vi "Yokogawa WT300 Series Measure Harmonics Preset.vi"() -> ()   [LabVIEW 2016]
doc: "This example shows how to measure the harmonic measurement numeric preset list data\n\n<b>Note:</b>\nThis setting valid on models with the harmonic measurement (/G5) option."
uses:
  Public/Data/Read Measurement (Harmonics).vi
  Yokogawa WT300 Series.lvlib
panel:
  in  "Preset (1:Pattern 1)":i32(ring)=1 items=["Pattern 1"=1, "Pattern 2"=2, "Pattern 3"=3, "Pattern 4"=4]
  out "Measurement":dbl[][](array[numeric])
  out "Function":string[](array[string])
  in  "Number of Item (15)":i32=15 min=1 max=32
  in  "Timeout (10000 ms)":i32=10000 min=1
  in  "VISA resource name":refnum<visa-resource-name>
  # "(c) 2013 Yokogawa Meters & Instruments Corporation.  All rights reserved."
  # "WT300 SERIES POWER ANALYZER"
  # "Total        DC            1             2              3             4"
  # "ms"
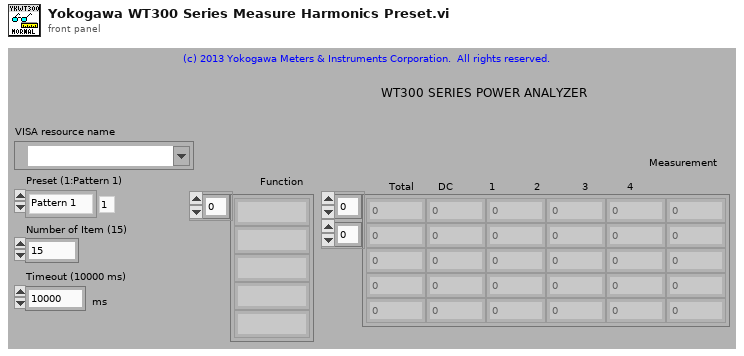
[diagram p1: front panel]
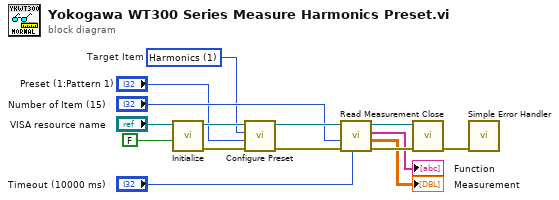
[diagram p0: block diagram]
diagram:
  w2 = 1 items=["Normal", "Harmonics"]  # Target Item
  n1 = call "Initialize.vi"("Reset (True)"=FALSE ("Reset? (True)"), "VISA resource name"="VISA resource name") -> ("error out"=w4:errorcluster, "VISA resource name out"=w5:refnum<visa-resource-name>)  [unwired: 7 in, 1 out]
  n2 = call "Configure Preset.vi"("error in (no error)"=w4, "Preset (1:Pattern 1)"="Preset (1:Pattern 1)", "Target Item (0: Normal)"=w2, "VISA resource name"=w5) -> ("error out"=w9:errorcluster, "VISA resource name out"=w10:refnum<visa-resource-name>)  [unwired: 6 in]
  n3 = call-poly "Read Measurement.vi"("Timeout (10000 ms)"="Timeout (10000 ms)", "error in (no error)"=w9, "Number of Item (15)"="Number of Item (15)", "VISA resource name"=w10) -> ("error out"=w12:errorcluster, "Measurement"=→"Measurement":dbl[][], "Function"=→"Function":string[], "VISA resource name out"=w13:refnum<visa-resource-name>)  [unwired: 4 in]
  n4 = call "Close.vi"("error in (no error)"=w12, "VISA resource name"=w13) -> ("error out"=w15:errorcluster)  [unwired: 9 in]
  n5 = call <vilib>:"Simple Error Handler.vi"("error in (no error)"=w15) -> ()  [unwired: 4 in, 5 out]
